vi "BotSpeakTCP_Init.vi"(1 "Bot Settings in":T1) -> (2 "error out":errorcluster, 3 "connection ID":refnum<k5>, 4 "Bot Settings out":T1)   [LabVIEW 2012]
uses:
  <userlib>/BotSpeak/VIs/Direct/BotSpeak_Control.ctl
  <userlib>/BotSpeak/VIs/SubVIs/BotSpeak_Globals.vi
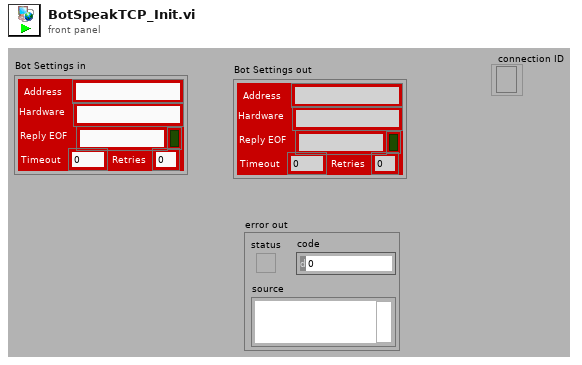
[diagram p1: front panel]
types:
  T1 = typedef "BotSpeak_Control.ctl" = cluster{"Address":string, "Reply EOF":string, "Hardware":string, "Retries":i8, "Timeout":i32, "Open?":bool}
  T2 = typedef "BotSpeak.HardwareSpecs.ctl" = cluster{"Hardware Name":string, "Hardware URL":string, "ComType":enum16{"Undefined", "Serial", "TCPIP", "Console", "EV3"}, "TCP Port":i32, "DefaultAddress":string, "Retries":i32, "Translate":enum16{"None", "Tiny", "URAPI"}, "MaxScriptSize":i32, "MaxVarNumber":i32, "StartupWait":i32, "Patience":i32, "Startup Patience":i32, "Hardware Help":string, "Com Protocol":string, "Translator":cluster{"BotSpeak CMD":string, "CMD out":string}[], "Init Code":string, "Variable Format":enum16{"INT", "FLOAT", "FIXED"}, "username":string, "password":string}
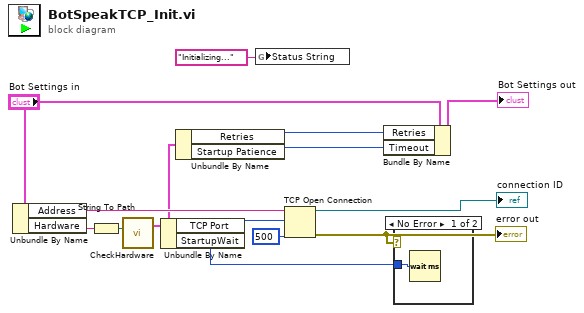
[diagram p0: block diagram]
diagram:
  n1 = Unbundle By Name("Bot Settings in") -> ("Address"=w14:string, "Hardware"=w11:string)
  n2 = String To Path(string=w11) -> (path=w1:path)
  n3 = call <userlib>:"CheckHardware.vi"("Hardware"=w1) -> ("HardwareSpecs"=w4:T2)  [unwired: 2 in]
  n4 = Unbundle By Name(w4) -> ("TCP Port"=w12:i32, "StartupWait"=w13:i32)
  n5 = Unbundle By Name(w4) -> ("Retries"=w3:i32, "Startup Patience"=w2:i32)
  n6 = global write "BotSpeak_Globals.vi" "Status String"("Initializing..." ("Status String")) -> ()
  n7 = TCP Open Connection(address=w14, remote port or service name=w12, timeout ms (60000)=500) -> (connection ID=→"connection ID":refnum<k5>, error out=w7:errorcluster)  [unwired: 2 in]
  "error out" <- w7
  n8 = Bundle By Name(cluster="Bot Settings in", "Retries"=w3, "Timeout"=w2) -> (→"Bot Settings out":T1)
  n9 = case shown="No Error" w7 {
    tunnel: w13 -> [w15 _]
    frame No Error {
      n10 = Wait (ms)(milliseconds to wait=w15) -> ()  [unwired: 1 out]
    }
    frame Error {
    }
  }
